vi "Read Save.vi"(8 "error in (no error)":errorcluster, 11 "Measurement Setup UI in":refnum<class "Measurement Setup UI.lvclass">) -> (0 "error out":errorcluster, 2 "Save":refnum<vi>, 3 "Measurement Setup UI out":refnum<class "Measurement Setup UI.lvclass">)   [LabVIEW 2017, in "Measurement Setup Controller.lvlib" / "Measurement Setup UI.lvclass"]
uses:
  Measurement Setup UI.lvclass
  Measurement Setup UI.lvclass/Measurement Setup UI.ctl
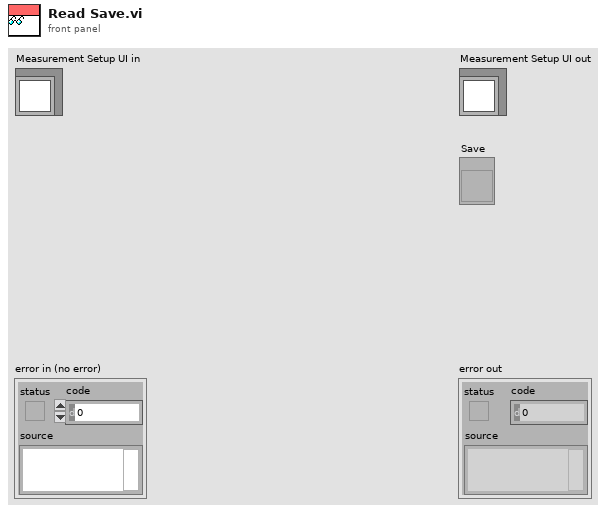
[diagram p1: front panel]
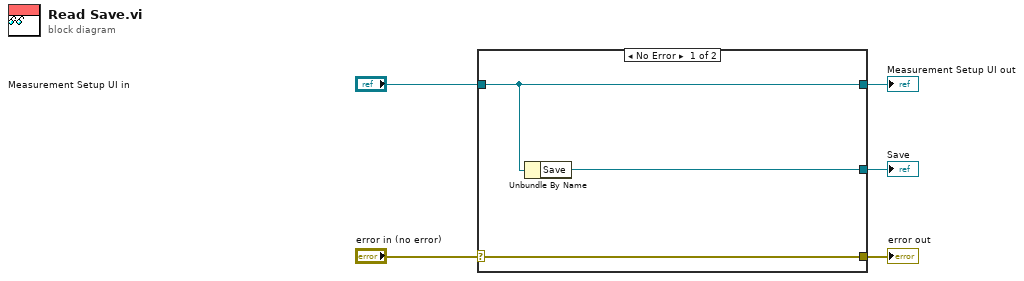
[diagram p0: block diagram]
diagram:
  n1 = case shown="No Error" "error in (no error)" {
    selector: "error in (no error)" -> [w8 w9]
    tunnel: [w8 w9] -> w4
    tunnel: [w7 w10] -> w2
    tunnel: "Measurement Setup UI in" -> [w7 w10]
    tunnel: [w6 _] -> w1
    frame No Error {
      n2 = Unbundle By Name(w7) -> ("Save"=w6:refnum<vi>)
    }
    frame Error {
    }
  }
  "error out" <- w4
  "Measurement Setup UI out" <- w2
  "Save" <- w1
